vi "test Undersized Destination Array.vi"(8 "error in (no error)":errorcluster, 11 "TestCase in":refnum<class "Malleable Tests.lvclass">) -> (0 "error out":errorcluster, 3 "TestCase out":refnum<class "Malleable Tests.lvclass">)   [LabVIEW 2020, in "Memory Manager Tests.lvlib" / "Malleable Tests.lvclass"]
uses:
  Malleable Tests.lvclass
  Malleable Type Tests/Malleable Type Tests.lvclass
  C:/dev/illuminated-g/labview-memory-management-tools/Source/Classes/Pointer/Pointer.lvclass
  4a897268-7aeb-4ca8-a05a-4b45b703c3ea.vi
  4a897268-7aeb-4ca8-a05a-4b45b703c3ea.vi/48144062-09e8-44d7-a914-3b058f1e4a5b.vi
  Source/Classes/Pointer/Write U64.vi
  Source/Classes/Pointer/Write U32.vi
  Source/Classes/Pointer/Write U16.vi
  Source/Classes/Pointer/Check Null Pointer.vi
  Source/Classes/Pointer/Get Size.vi
  Source/Classes/Pointer/Get Address.vi
  Source/Classes/Pointer/Errors.vi
  Source/Classes/Pointer/Out of Bounds.vi
  <vilib>/addons/_JKI Toolkits/VI Tester/TestCase.llb/TestCase.lvclass
  Source/Classes/Pointer/Pointer.lvclass
  C:/dev/illuminated-g/labview-memory-management-tools/Tests/Memory Manager/Malleable Type Tests/Malleable Type Tests.lvclass
  C:/Program Files (x86)/National Instruments/LabVIEW 2020/vi.lib/addons/_JKI Toolkits/VI Tester/TestCase.llb/TestCase.lvclass
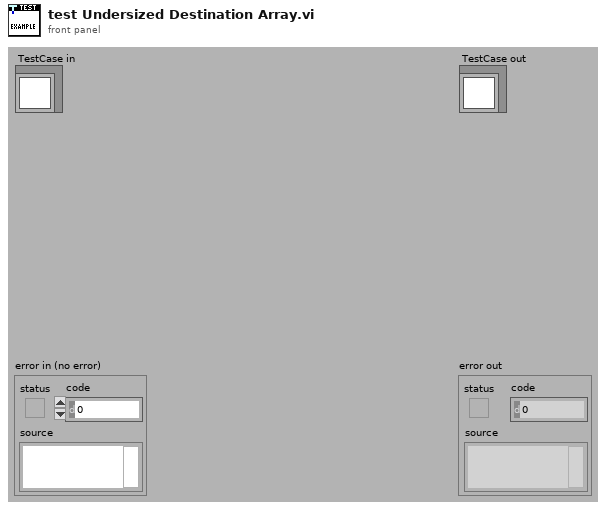
[diagram p1: front panel]
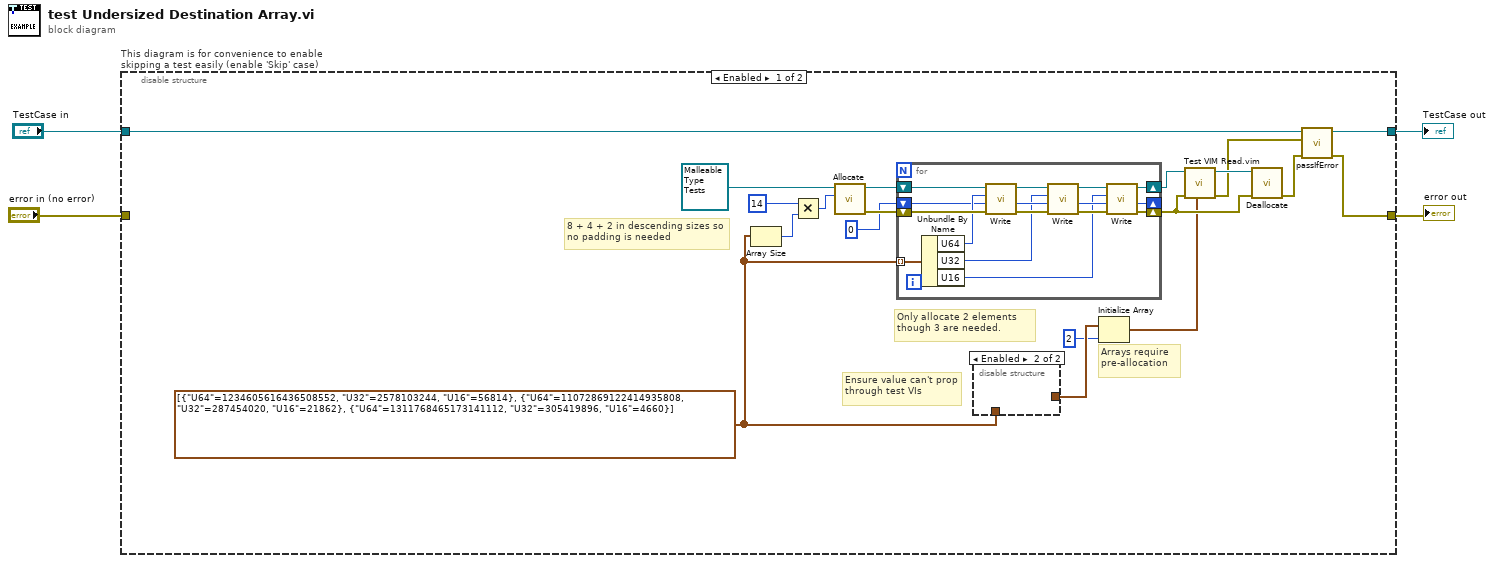
[diagram p0: block diagram]
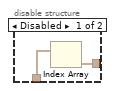
[diagram p2: hidden frame]
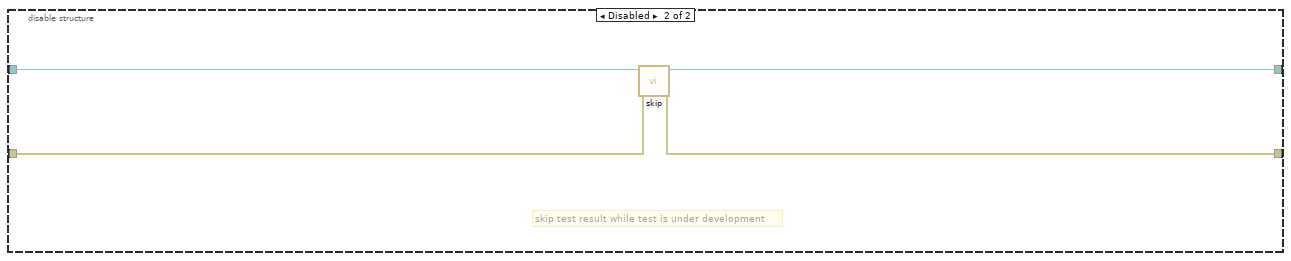
[diagram p3: hidden frame]
diagram:
  n1 = disable-structure "This diagram is for convenience to enable skipping a test easily (enable 'Skip' case)" shown="Enabled" {
    disable-tunnel: "TestCase in" -> [w8 w45]
    disable-tunnel: [w9 w43] -> w1
    disable-tunnel: [w5 w44] -> w3
    disable-tunnel: "error in (no error)" -> [_ w42]
    frame Enabled {
      w14 = cluster{"U64":u64, "U32":u32, "U16":u16}[] [{"U64"=1234605616436508552, "U32"=2578103244, "U16"=56814}, {"U64"=11072869122414935808, "U32"=287454020, "U16"=21862}, {"U64"=1311768465173141112, "U32"=305419896, "U16"=4660}]
      # "Only allocate 2 elements though 3 are needed."
      # "Arrays require pre-allocation"
      # "Ensure value can't prop through test VIs"
      # "8 + 4 + 2 in descending sizes so no padding is needed"
      n2 = Array Size(array=w14) -> (size(s)=w11:i32)
      n3 = Multiply(x=u64 14 ("size"), y=w11) -> (x*y=w15:u64)
      n4 = call "Allocate.vi"("size"=w15, "Pointer type"=refnum<class "Malleable Type Tests.lvclass"> refnum ("Memory Manager Tests.lvlib:Malleable Type Tests.lvclass")) -> ("error out"=w19:errorcluster, "Pointer out"=w20:refnum<class "Malleable Type Tests.lvclass">)  [unwired: 8 in]
      n5 = for {
        shift-right: [w28] -> w18
        shift-left: w20 -> [w39]
        shift-right: [w27] -> w23
        shift-left: w19 -> [w38]
        tunnel: w14 -> [w26] mode=indexing
        shift-right: [w25] -> _
        shift-left: u64 0 ("offset + size") -> [w24]
        n6 = Unbundle By Name(w26) -> ("U64"=w37:u64, "U32"=w33:u32, "U16"=w29:u16)
        n7 = call-poly "Write.vi"("error in (no error)"=w38, "offset (0)"=w24, "value"=w37, "Pointer in"=w39) -> ("error out"=w35:errorcluster, "offset + size"=w34:u64, "Pointer out"=w36:refnum<class "Malleable Type Tests.lvclass">)  [unwired: 4 in, 1 out]
        n8 = call-poly "Write.vi"("error in (no error)"=w35, "offset (0)"=w34, "value"=w33, "Pointer in"=w36) -> ("error out"=w31:errorcluster, "offset + size"=w30:u64, "Pointer out"=w32:refnum<class "Malleable Type Tests.lvclass">)  [unwired: 4 in, 1 out]
        n9 = call-poly "Write.vi"("error in (no error)"=w31, "offset (0)"=w30, "value"=w29, "Pointer in"=w32) -> ("error out"=w27:errorcluster, "offset + size"=w25:u64, "Pointer out"=w28:refnum<class "Malleable Type Tests.lvclass">)  [unwired: 4 in, 1 out]
      }
      n10 = disable-structure shown="Enabled" {
        disable-tunnel: w14 -> [w41 _]
        disable-tunnel: [w40 _] -> w17
        frame Disabled {
          n11 = Index Array(array=w41) -> (element=w40:cluster{"U64":u64, "U32":u32, "U16":u16})  [unwired: 1 in]
        }
        frame Enabled {
        }
      }
      n12 = Initialize Array(w17, 2 ("dimension size")) -> (w12:cluster{"U64":u64, "U32":u32, "U16":u16}[])
      n13 = call "Test VIM Read.vim"("Type"=w12, "error in (no error)"=w23, "Malleable Type Tests in"=w18) -> ("error out"=w7:errorcluster, "Malleable Type Tests out"=w16:refnum<class "Malleable Type Tests.lvclass">)  [unwired: 6 in, 1 out]
      n14 = call "Deallocate.vi"("error in (no error)"=w23, "Pointer"=w16) -> ("error out"=w6:errorcluster)  [unwired: 8 in, 1 out]
      n15 = call-dynamic "passIfError.vi"("error in (no error)"=w6, "error"=w7, "TestCase in"=w8) -> ("error out"=w5:errorcluster, "TestCase out"=w9:refnum<class "Malleable Tests.lvclass">)  [unwired: 7 in]
    }
    frame Disabled {
      # "skip test result while test is under development"
      n16 = call <vilib>:"skip.vi"("error in (no error)"=w42, "TestCase in"=w45) -> ("error out"=w44:errorcluster, "TestCase out"=w43:refnum<class "Malleable Tests.lvclass">)  [unwired: 8 in]
    }
  }
  "error out" <- w3
  "TestCase out" <- w1
